vi "MQTT Transmitter (DBL).vi"() -> ()   [LabVIEW 2021]
uses:
  <vilib>/LabVIEW Open Source Project/MQTT Control Packets/Control Packets/CONNECT/ConnectFlags -- cluster.ctl
  <vilib>/LabVIEW Open Source Project/MQTT Client/Client class/Client.lvclass/Client.ctl
  <vilib>/LabVIEW Open Source Project/MQTT Client/Client class/Client.lvclass
  C:/Program Files (x86)/National Instruments/LabVIEW 2021/vi.lib/LabVIEW Open Source Project/MQTT Connection/MQTT_Base/Base Class/MQTT_Base.lvclass
  <vilib>/LabVIEW Open Source Project/Connection/Connection.TCP/Connection.TCP.lvclass
  C:/Program Files (x86)/National Instruments/LabVIEW 2021/vi.lib/LabVIEW Open Source Project/Connection/Connection/Connection.lvclass
  <vilib>/LabVIEW Open Source Project/MQTT Control Packets/Control Packets/PUBLISH/PUBLISH.lvclass
  <vilib>/LabVIEW Open Source Project/MQTT Connection/MQTT_Base/Base Class/MQTT_Base.lvclass
  <vilib>/LabVIEW Open Source Project/MQTT Control Packets/Control Packets/CONNECT/CONNECT.lvclass
panel:
  out "Published":bool
  in  "Send Topic":string="other/string"
  out "Send Chart":dbl(graph)
  out "Data Send":dbl format="%#_4g"
  in  "Time Target (s)":dbl=0.1 format="%#_6ps"
  out "Connected?":bool
  out "Read Chart":dbl(graph)
  out "Data Read":dbl format="%#_4g"
  in  "Read Topic":string="some/string"
  in  "remote port (1883)":u16=1883
  in  "address (localhost)":string="localhost"
  in  "STOP":bool
  # "MQTT Transmitter"
  # "Read"
  # "Send"
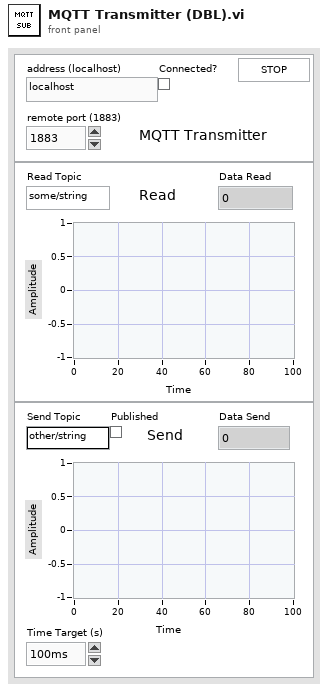
[diagram p1: front panel]
types:
  T1 = enum32{"Invalid", "Standard", "Closed", "Hidden", "Minimized", "Maximized"}
  T2 = enum32{"invalid app kind", "Development System", "Run Time System", "Student Edition", "Embedded LabVIEW", "Evaluation", "Custom"}
  T3 = cluster{"Will Topic":string, "Will Message":string, "Username":string, "Password":string}
  T4 = typedef "MQTT_Control_Packets.lvlib/CONNECT.lvclass/ConnectFlags -- cluster.ctl" = cluster{"Reserved":bool, "Clean Session":bool, "Will Flag":bool, "Will QoS 1":bool, "Will QoS 2":bool, "Will Retain":bool, "Password Flag":bool, "User Name Flag":bool}
  T5 = cluster{"Core":cluster{"Current VI Reference":refnum<vi>, "Close Panel on Exit?":bool}, "Connected?":bool, "Published?":bool, "Dummy Data":dbl}
  T6 = cluster{"Current VI Reference":refnum<vi>, "Close Panel on Exit?":bool}
  T7 = typedef "MQTT Client.lvlib/Client.lvclass/Public Events -- cluster.ctl" = cluster{"Connection Status":refnum<user-event>, "Connected":refnum<user-event>, "Application Message":refnum<user-event>}
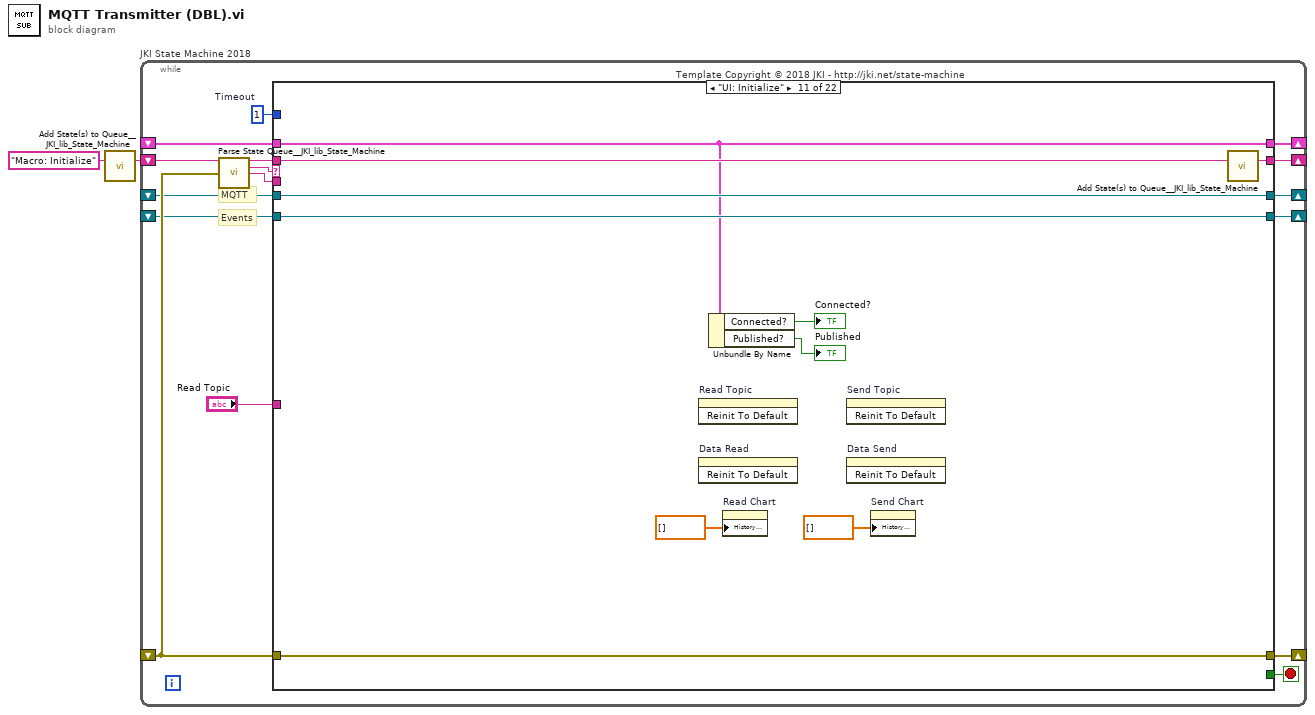
[diagram p0: block diagram]
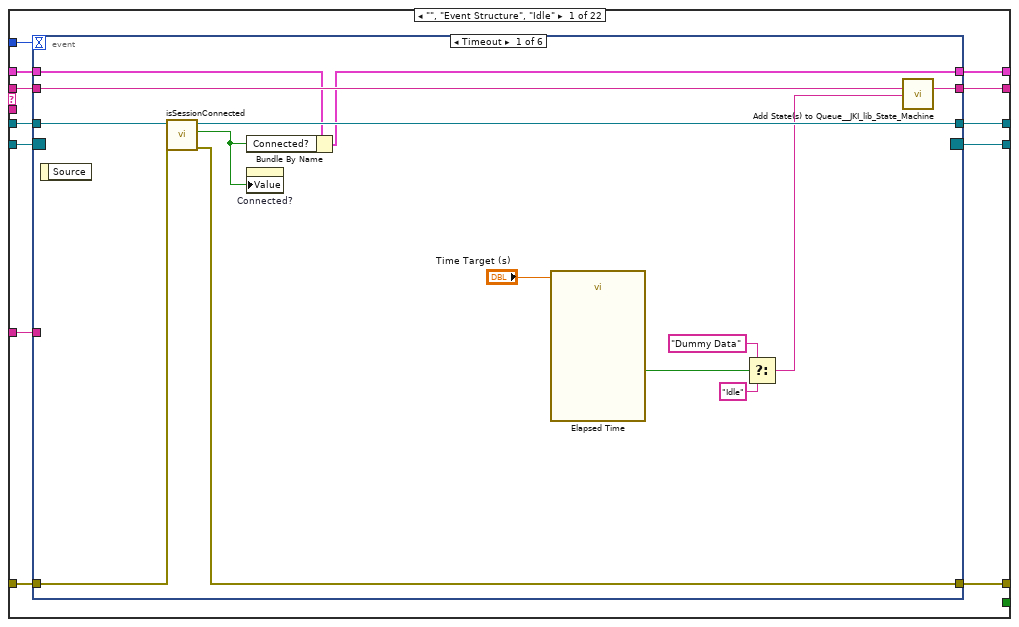
[diagram p2: hidden frame]
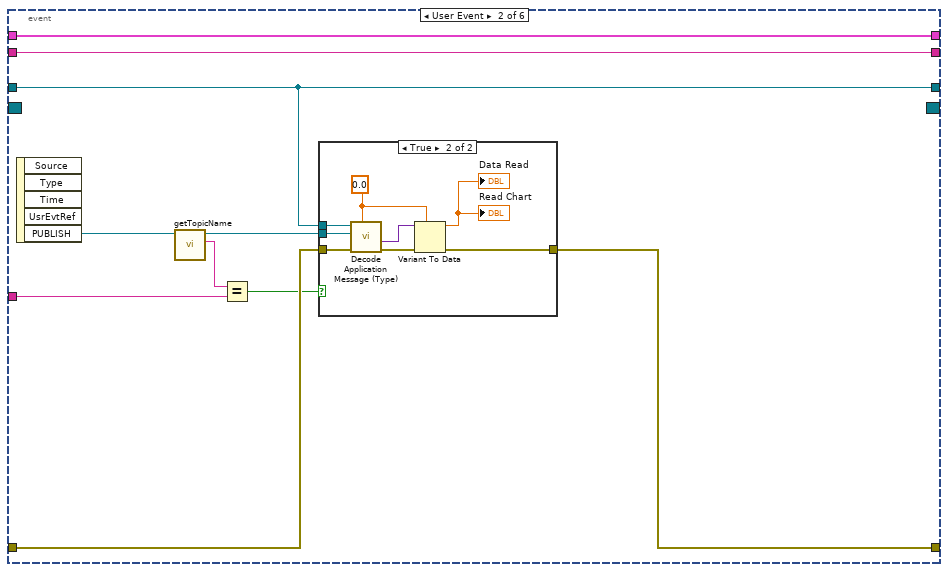
[diagram p3: hidden frame]
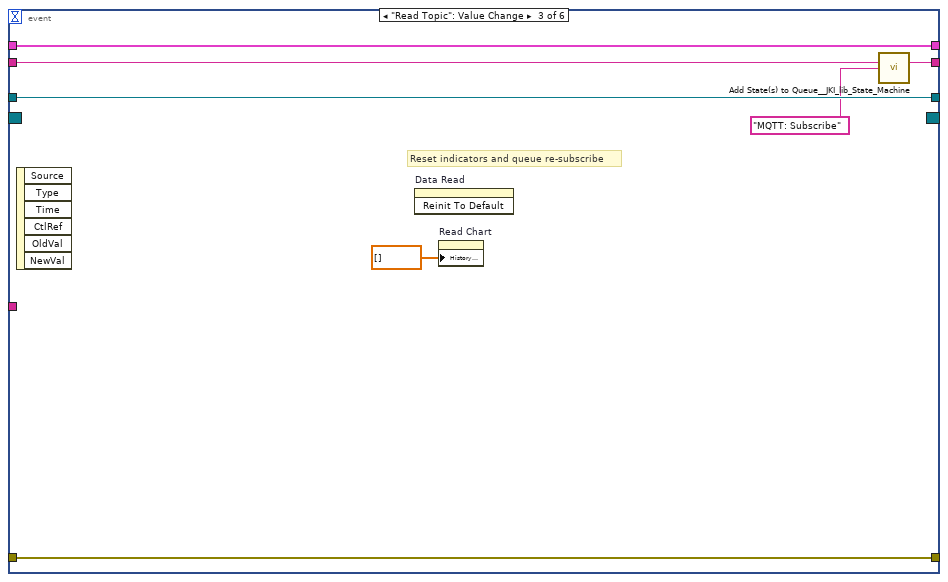
[diagram p5: hidden frame]
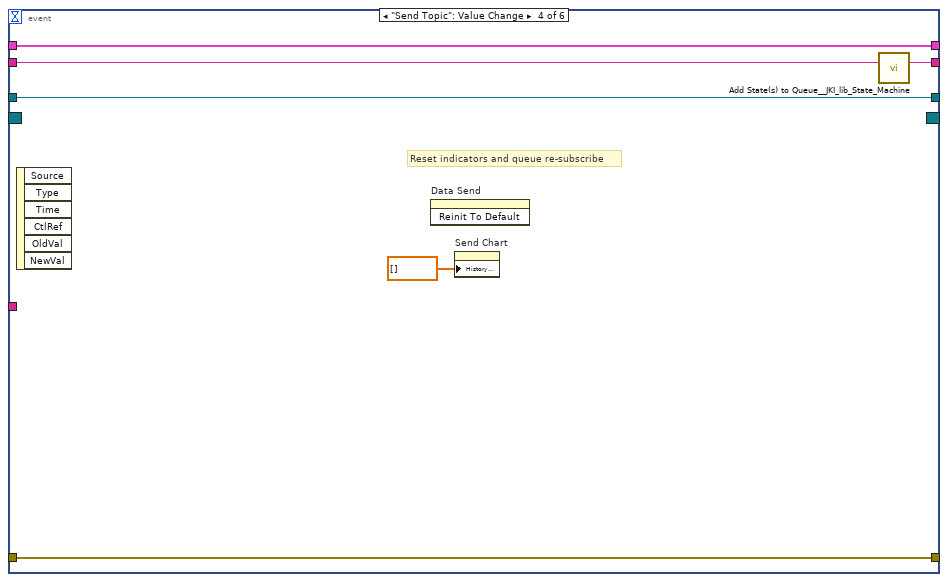
[diagram p6: hidden frame]
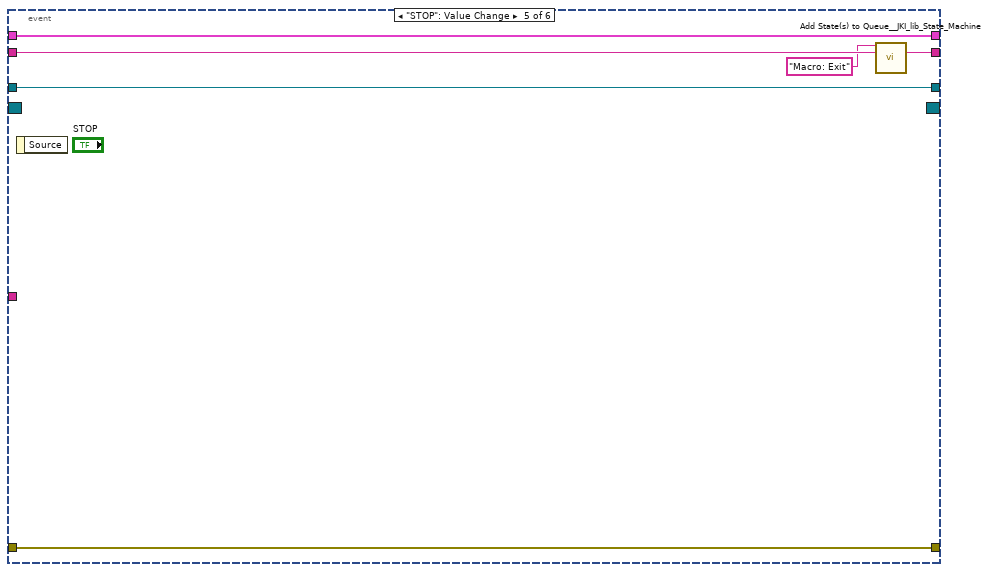
[diagram p7: hidden frame]
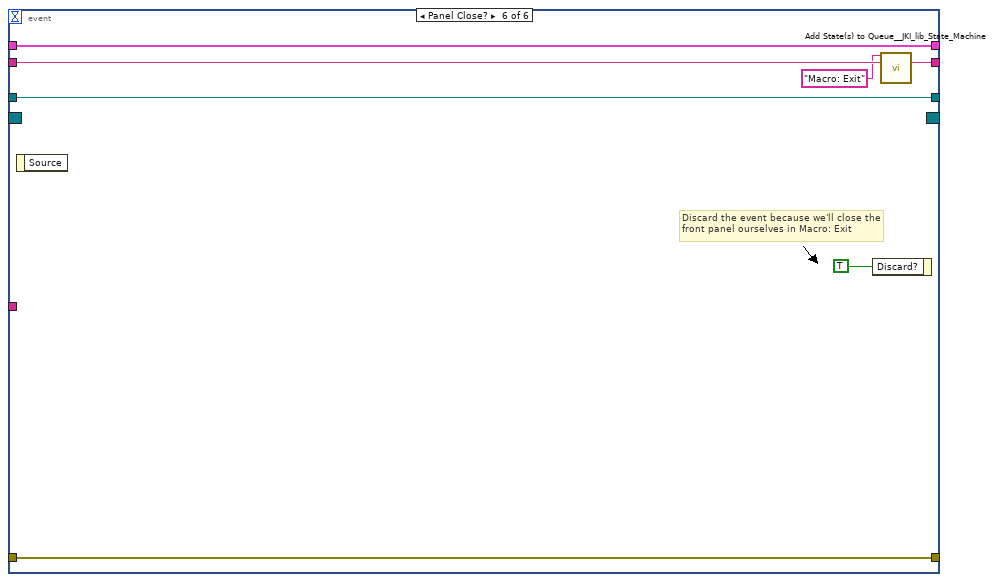
[diagram p8: hidden frame]
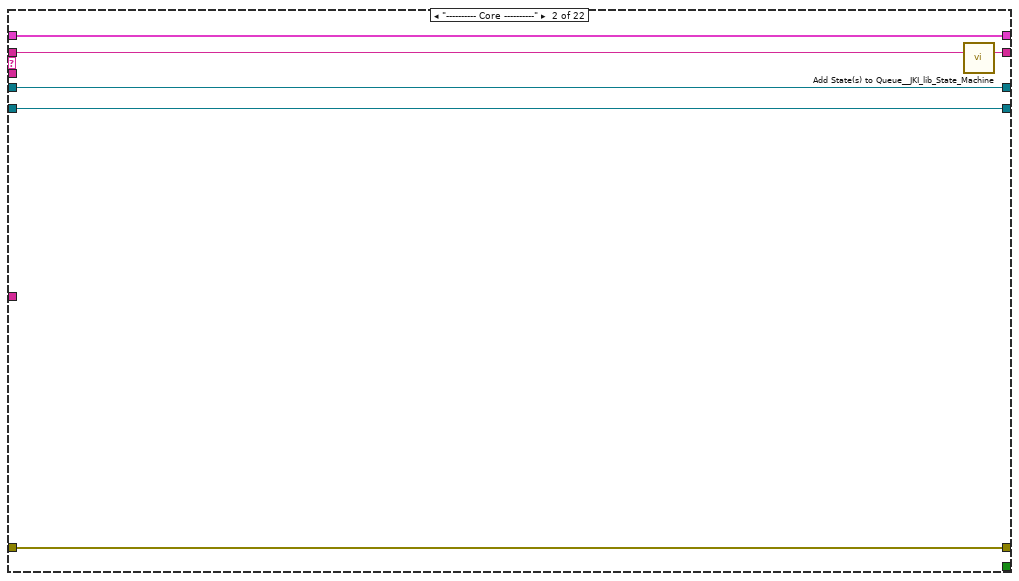
[diagram p9: hidden frame]
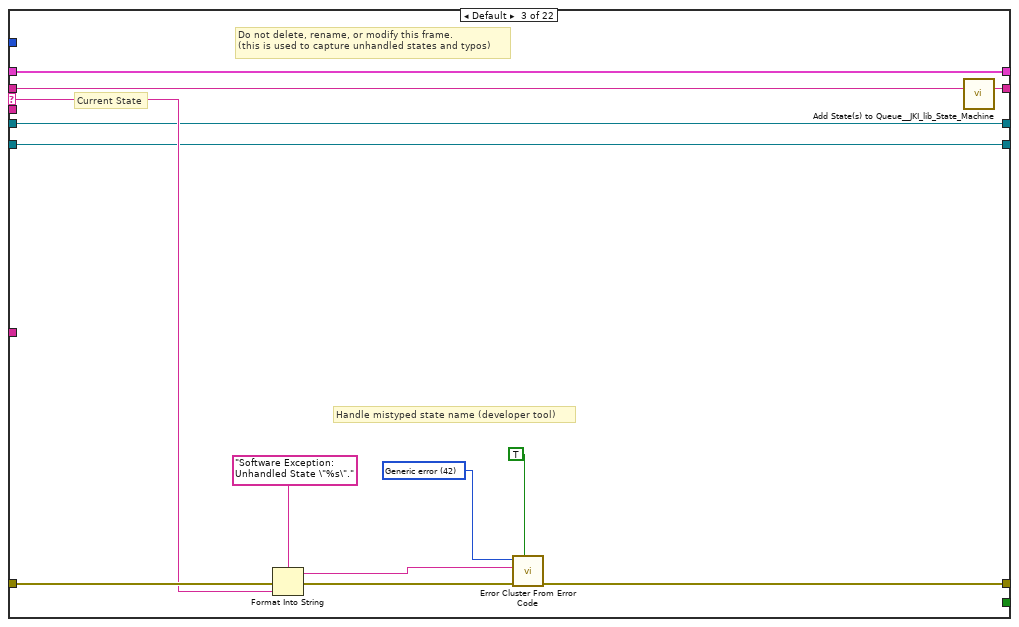
[diagram p10: hidden frame]
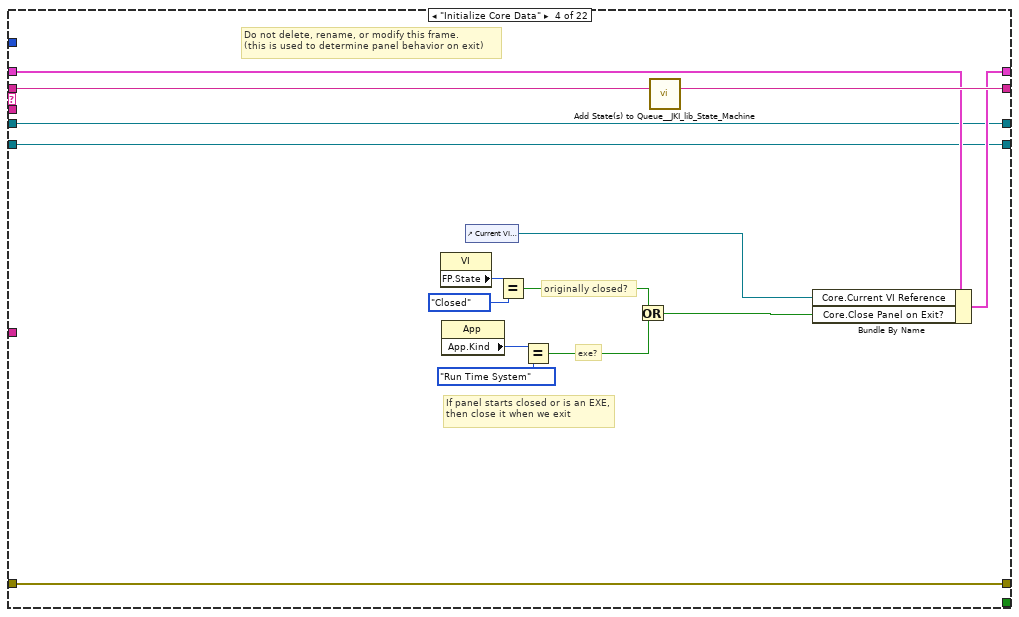
[diagram p11: hidden frame]
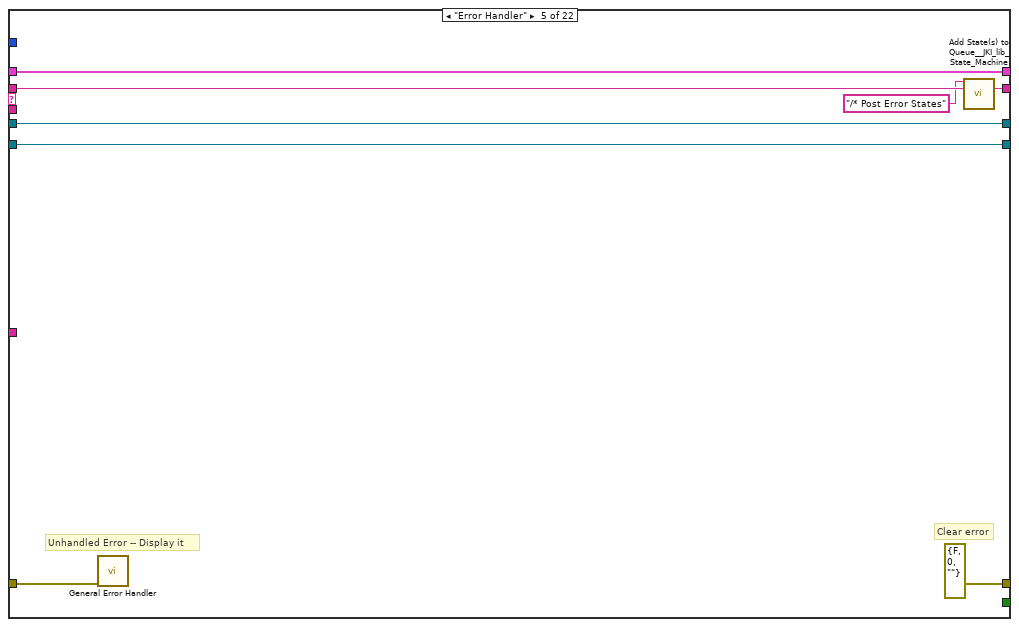
[diagram p12: hidden frame]
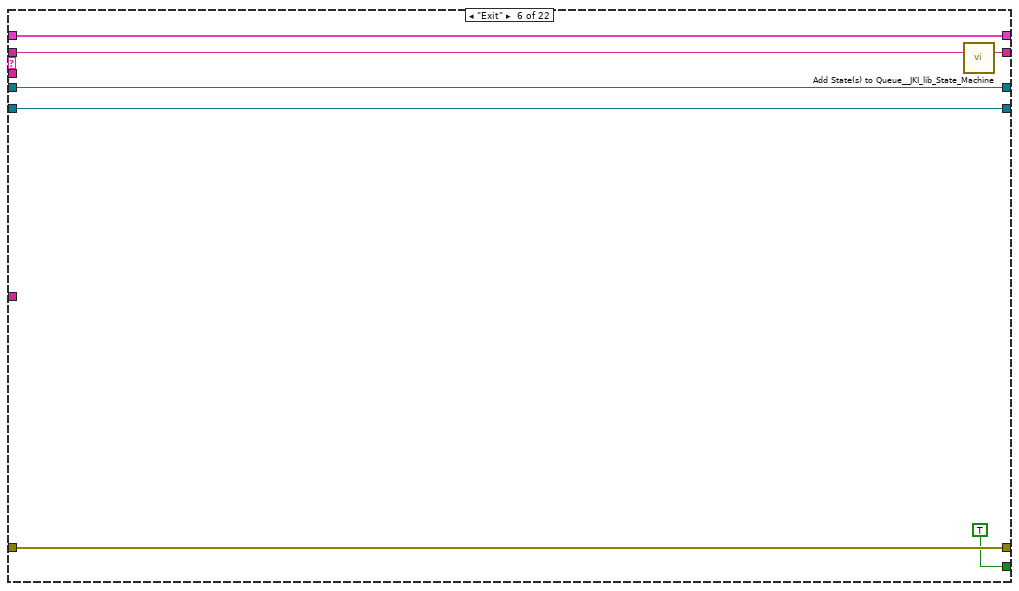
[diagram p13: hidden frame]
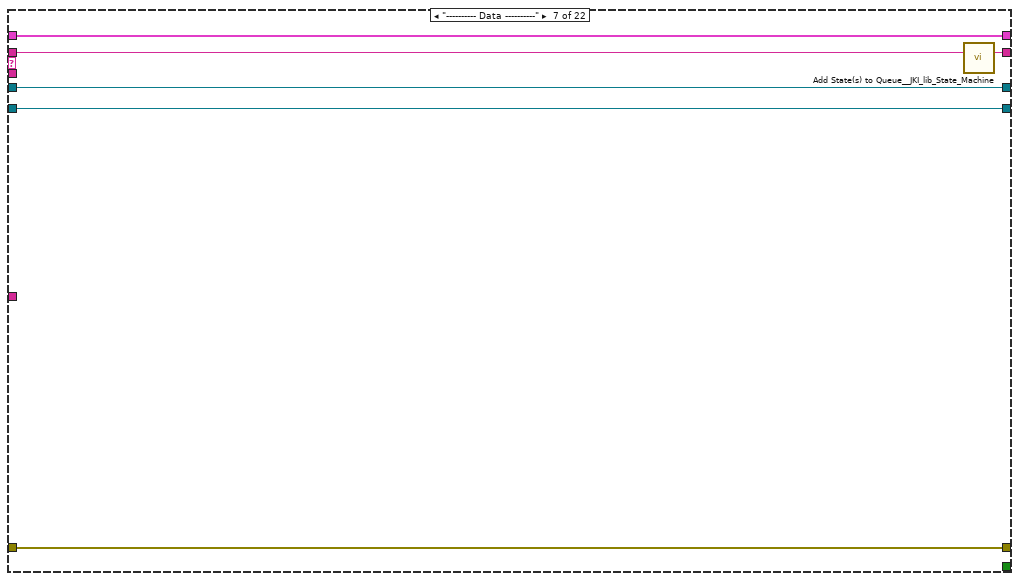
[diagram p14: hidden frame]
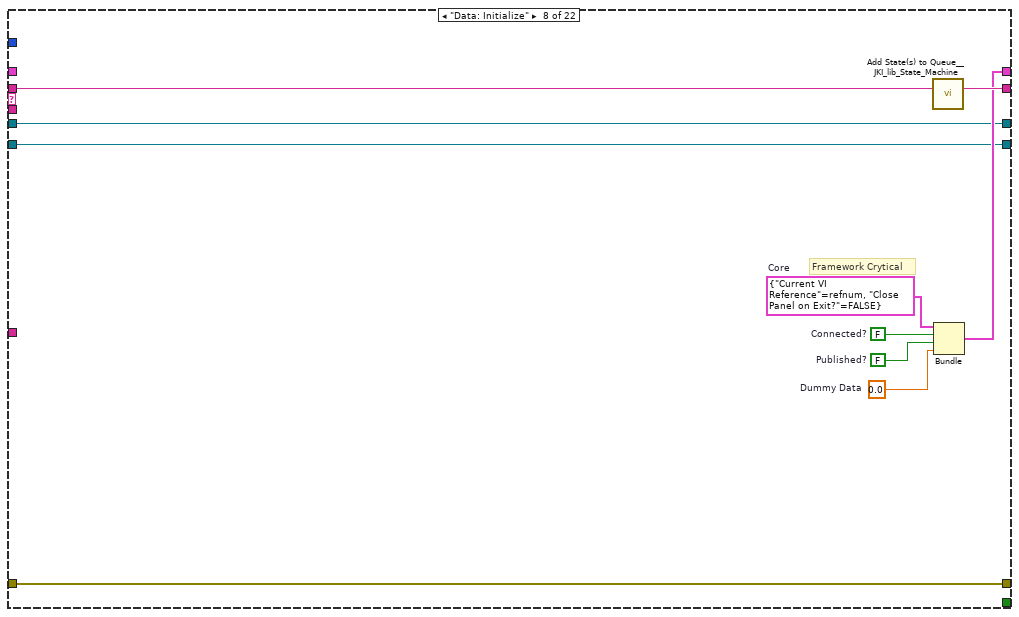
[diagram p15: hidden frame]
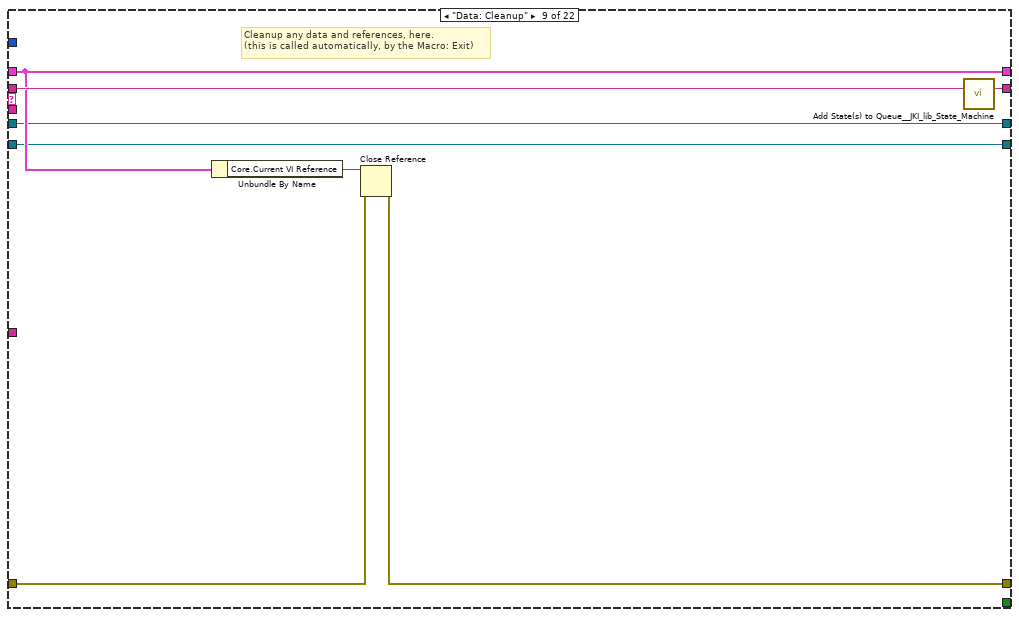
[diagram p16: hidden frame]
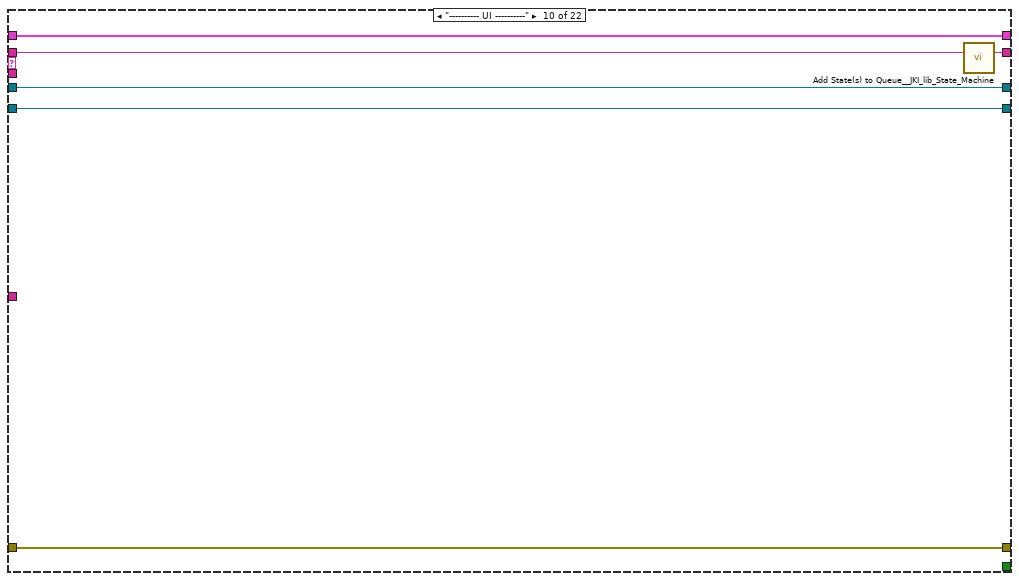
[diagram p17: hidden frame]
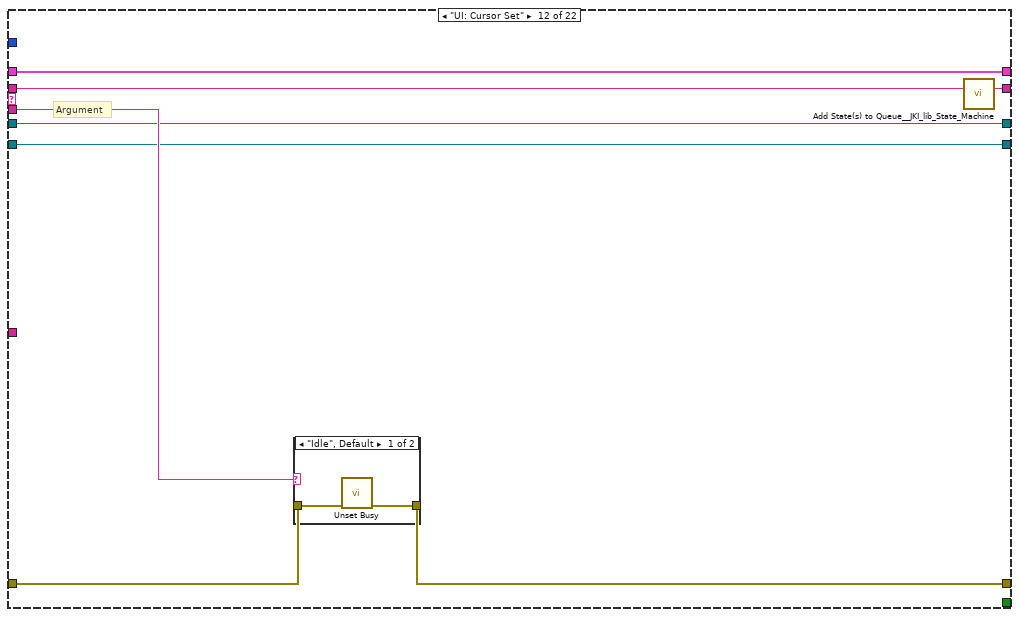
[diagram p18: hidden frame]
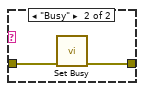
[diagram p19: hidden frame]
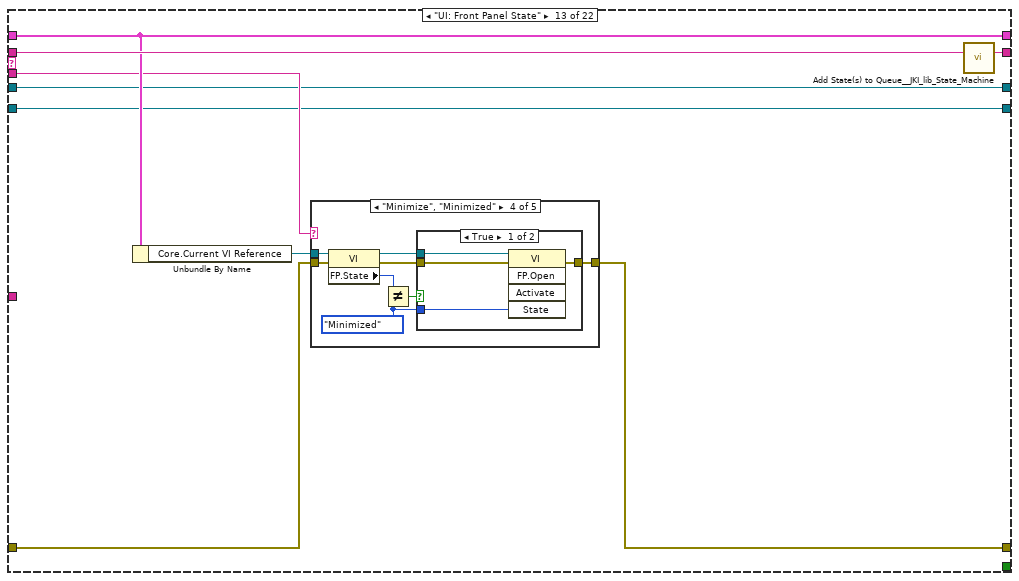
[diagram p20: hidden frame]
diagram:
  n1 = call <vilib>:"Add State(s) to Queue__JKI_lib_State_Machine.vi"("State(s) in (\"\")"="Macro: Initialize") -> ("States Out"=w2:string)  [unwired: 14 in]
  n2 = while "JKI State Machine 2018" {
    shift-right: [w11] -> _
    shift-left: _ -> [w10]
    shift-right: [w14] -> _
    shift-left: _ -> [w8]
    shift-right: [w13] -> _
    shift-left: w2 -> [w15]
    shift-right: [w7] -> _
    shift-left: _ -> [w6]
    shift-right: [w5] -> _
    shift-left: _ -> [w4]
    stop <- w12 stop-if-true
    w9 = 1  # Timeout
    # "Events"
    # "MQTT"
    # "Template Copyright © 2018 JKI - http://jki.net/state-machine"
    n3 = call <vilib>:"Parse State Queue__JKI_lib_State_Machine.vi"("State Queue"=w15, "Error In (no error)"=w8) -> ("Remaining States"=w17:string, "Current State"=w18:string, "Arguments"=w16:string)  [unwired: 11 in]
    n4 = case shown="\"UI: Initialize\"" w18 {
      selector: w18 -> [_ _ w98 _ _ _ _ _ _ _ _ _ _ _ _ _ _ _ _ _ _ _]
      tunnel: w17 -> [w30 w95 w102 w123 w131 w138 w144 w154 w162 w168 w178 w186 w199 w270 w277 w289 w295 w323 w325 w344 w364 w373]
      tunnel: w16 -> [_ _ _ _ _ _ _ _ _ _ _ w181 w193 _ _ _ _ _ _ _ _ _]
      tunnel: w10 -> [w28 w92 w100 w116 w128 w136 w141 _ w157 w165 w173 w184 w195 w267 w274 w286 w292 w303 w324 w342 w366 w371]
      tunnel: [w27 w93 w104 w120 errorcluster {"status"=FALSE, "code"=0, "source"=""} ("error out") w135 w142 w151 w158 w166 w176 w182 w196 w268 w275 w287 w293 w305 w326 w345 w365 w372] -> w14
      tunnel: w8 -> [w26 w93 w103 w120 w127 w135 w142 w151 w159 w166 w176 w183 w197 w268 w275 w287 w293 w321 w327 w348 w365 w372]
      tunnel: [w29 w94 w101 w122 w130 w137 w143 w153 w161 w167 w177 w185 w198 w269 w276 w288 w294 w322 w325 w344 w364 w375] -> w13
      tunnel: [_ _ _ _ _ TRUE _ _ _ _ _ _ _ _ _ _ _ _ _ _ _ _] -> w12
      tunnel: [w25 w92 w100 w121 w128 w136 w141 w152 w157 w165 w173 w184 w195 w267 w274 w286 w292 w302 w324 w343 w366 w370] -> w11
      tunnel: w9 -> [w24 _ _ _ _ _ _ _ _ _ _ _ _ _ _ _ _ _ _ _ _ _]
      tunnel: [w20 w90 w96 w109 w124 w132 w139 w147 w155 w163 w174 w179 w191 w265 w271 w278 w290 w320 w334 w353 w368 w378] -> w7
      tunnel: w6 -> [w21 w90 w96 w109 w124 w132 w139 w147 w155 w163 w174 w179 w191 w265 w271 w278 w290 _ w334 w353 w368 w378]
      tunnel: [w22 w91 w97 w110 w125 w133 w140 w148 w156 w164 w175 w180 w192 w266 w272 w279 w291 w304 w328 w346 w367 w377] -> w5
      tunnel: w4 -> [w23 w91 w97 w110 w125 w133 w140 w148 w156 w164 w175 w180 w192 w266 w272 w279 w291 _ w329 w347 w367 w377]
      tunnel: "Read Topic" -> [w19 _ _ _ _ _ _ _ _ _ _ _ _ _ _ _ _ _ w330 _ _ _]
      frame "", "Event Structure", "Idle" {
        n5 = event shown="[0] Timeout" {
          selector: w21 -> [_ _ _ _ _ _]
          dyn-events: [_ _ _ _ _ _] -> w20
          timeout: w24 -> [_ _ _ _ _ _]
          tunnel: w30 -> [w44 w54 w69 w75 w82 w89]
          tunnel: [w43 w54 w68 w74 w81 w88] -> w29
          tunnel: w28 -> [w38 w53 w70 w76 w79 w86]
          tunnel: [w39 w48 w67 w73 w80 w87] -> w27
          tunnel: w26 -> [w40 w49 w67 w73 w80 w87]
          tunnel: [w37 w53 w70 w76 w79 w86] -> w25
          tunnel: w23 -> [w42 w50 w66 w72 w77 w83]
          tunnel: [w41 w50 w66 w72 w77 w83] -> w22
          tunnel: w19 -> [_ w51 _ _ _ _]
          event Timeout {
            n6 = event-data() -> ()  [unwired: 1 in, 1 out]
            n7 = call <vilib>:"isSessionConnected.vi"("error in (no error)"=w40, "MQTT_Base in"=w42) -> ("error out"=w39:errorcluster, "Connected?"=w36:bool, "MQTT_Base out"=w41:refnum<class "Client.lvclass">)  [unwired: 7 in]
            n8 = Bundle By Name(cluster=w38, "Connected?"=w36) -> (w37:T5)
            n9 = property on="Connected?" class="Bool (strict)"("Value"=w36) -> ()  [unwired: 2 in, 2 out]
            n10 = call "Elapsed Time"("Time Target (s)"="Time Target (s)") -> ("Time has Elapsed"=w35:bool)  [unwired: 11 in, 7 out]
            n11 = Select(t="Dummy Data" ("State(s) at Back (\"\")"), s=w35, f="Idle" ("State(s) at Back (\"\")")) -> (s? t:f=w32:string)
            n12 = call <vilib>:"Add State(s) to Queue__JKI_lib_State_Machine.vi"("State(s) in (\"\")"=w44, "State(s) at Back (\"\")"=w32) -> ("States Out"=w43:string)  [unwired: 13 in]
          }
          event User Event {
            n13 = event-data() -> ("PUBLISH"=w52:refnum<class "PUBLISH.lvclass">)  [unwired: 1 in, 4 out]
            n14 = call <vilib>:"getTopicName.vi"("PUBLISH in"=w52) -> ("Topic"=w45:string, "PUBLISH out"=w46:refnum<class "PUBLISH.lvclass">)  [unwired: 8 in, 1 out]
            n15 = Equal?(x=w45, y=w51) -> (x = y?=w47:bool)
            n16 = case shown="True" w47 {
              tunnel: w50 -> [_ w63]
              tunnel: w49 -> [w55 w62]
              tunnel: [w55 w57] -> w48
              tunnel: w46 -> [_ w56]
              frame False {
              }
              frame True {
                w59 = 0.0
                n17 = call <vilib>:"Decode Application Message (Type).vi"("Type"=w59, "error in (no error)"=w62, "PUBLISH"=w56, "Client in"=w63) -> ("error out"=w60:errorcluster, "Payload"=w61:variant)  [unwired: 4 in, 2 out]
                n18 = Variant To Data(error in=w60, type=w59, Variant=w61) -> (data=→"Data Read" →"Read Chart":dbl, error out=w57:errorcluster)
              }
            }
          }
          event "Read Topic": Value Change {
            # "Reset indicators and queue re-subscribe"
            n19 = event-data() -> ()  [unwired: 1 in, 6 out]
            n20 = invoke on="Data Read" class="DigNum (strict)" method="Reinit To Default"() -> ()  [unwired: 3 in, 3 out]
            n21 = property on="Read Chart" class="WFChart (strict)"("History Data"=dbl[] []) -> ()  [unwired: 2 in, 2 out]
            n22 = call <vilib>:"Add State(s) to Queue__JKI_lib_State_Machine.vi"("State(s) in (\"\")"=w69, "State(s) at Back (\"\")"="MQTT: Subscribe" ("State(s) at Back (\"\")")) -> ("States Out"=w68:string)  [unwired: 13 in]
          }
          event "Send Topic": Value Change {
            # "Reset indicators and queue re-subscribe"
            n23 = event-data() -> ()  [unwired: 1 in, 6 out]
            n24 = invoke on="Data Send" class="DigNum (strict)" method="Reinit To Default"() -> ()  [unwired: 3 in, 3 out]
            n25 = property on="Send Chart" class="WFChart (strict)"("History Data"=dbl[] []) -> ()  [unwired: 2 in, 2 out]
            n26 = call <vilib>:"Add State(s) to Queue__JKI_lib_State_Machine.vi"("State(s) in (\"\")"=w75) -> ("States Out"=w74:string)  [unwired: 14 in]
          }
          event "STOP": Value Change {
            n27 = event-data() -> ()  [unwired: 1 in, 1 out]
            n28 = call <vilib>:"Add State(s) to Queue__JKI_lib_State_Machine.vi"("State(s) in Front (\"\")"="Macro: Exit", "State(s) in (\"\")"=w82) -> ("States Out"=w81:string)  [unwired: 13 in]
          }
          event Panel Close? {
            # "Discard the event because we'll close the front panel ourselves in Macro: Exit"
            n29 = event-data() -> ()  [unwired: 1 in, 1 out]
            n30 = event-data("Discard?"=TRUE) -> ()  [unwired: 1 in, 1 out]
            n31 = call <vilib>:"Add State(s) to Queue__JKI_lib_State_Machine.vi"("State(s) in Front (\"\")"="Macro: Exit", "State(s) in (\"\")"=w89) -> ("States Out"=w88:string)  [unwired: 13 in]
          }
        }
      }
      frame "---------- Core ----------" {
        n32 = call <vilib>:"Add State(s) to Queue__JKI_lib_State_Machine.vi"("State(s) in (\"\")"=w95) -> ("States Out"=w94:string)  [unwired: 14 in]
      }
      frame Default {
        w107 = 42 items=["No error", "Argument error", "Memory is full", "Out of zone", "End of file", "File already open", "Generic file I/O error", "File not found", "File permission error", "Disk is full", "Duplicate path", "Too many files open", "System feature not enabled", "Resource file not found", "Cannot add resource", "Resource not found", "Image not found", "Image memory error", "Pen does not exist", "Config type invalid", "Config token not found", "Config parse error", "Config memory error", "Bad external code format", "Bad external code offset", "External code not present", "Null window", "Destroy window error", "Null menu", "Print aborted", "Bad print record", "Print driver error", "Windows error during printing", "Memory error during printing", "Print dialog error", "Generic print error", "Invalid device refnum", "Device not found", "Device parameter error", "Device unit error", "Cannot open device", "Device call aborted", "Generic error", "Cancelled by user", "Object ID too low", "Object ID too high", "Object not in heap", "Unknown heap", "Unknown object (invalid DefProc)", "Unknown object (DefProc not in table)", "Message out of range", "Invalid (null) method", "Unknown message", "Manager call not supported", "Bad address", "Network operation in progress", "Network operation timed out", "Connection is busy", "Network attribute not supported", "Network error", "Address in use", "System out of memory", "Connection aborted", "Connection refused", "Not connected", "Already connected", "Connection closed", "Initialization error (interapplication manager)", "Bad occurrence", "Wait on unbound occurrence handler", "Occurrence queue overflow", "Datalog type conflict", "Unused", "Unrecognized type (interapplication manager)", "Memory corrupt", "Failed to make temporary DLL", "Old CIN version", "Drag socket not found", "Failed to load drop-object", "Failed to register OLE object", "Failed to release OLE object", "Format specifier type mismatch", "Unknown format specifier", "Too few format specifiers", "Too many format specifiers", "Scan failed", "Newer CIN version", "Error converting to variant", "Runtime menu error", "Password tampered", "Variant attribute not found", "Incompatible variant data type", "Event data is not available", "Event Store is not present", "Occurrence is not found", "Event Queue is not created", "Event info is not available", "Refnum passed is NULL", "Error retrieving Class GUID", "Error retrieving CoClass GUID", "Error retrieving TypeLib GUID.", "Bad built application magic bytes.", "Specific driver is different from the specific driver associated with the Logical Name.", "There is no session opened to the class driver.", "Max Error", "MAX - Error with config objects", "MAX - Error loading configuration", "MAX - Group not supported"]
        # "Current State"
        # "Do not delete, rename, or modify this frame.\n(this is used to capture unhandled states and typos)"
        # "Handle mistyped state name (developer tool)"
        n33 = Format Into String(format string="Software Exception: Unhandled State \"%s\"." ("message"), error in=w103, w98) -> (resulting string=w106:string, error out=w105:errorcluster)  [unwired: 1 in]
        n34 = call <vilib>:"Error Cluster From Error Code.vi"("show call chain? (False)"=TRUE, "error in (no error)"=w105, "error message (\"\")"=w106, "error code (0)"=w107) -> ("error out"=w104:errorcluster)  [unwired: 5 in]
        n35 = call <vilib>:"Add State(s) to Queue__JKI_lib_State_Machine.vi"("State(s) in (\"\")"=w102) -> ("States Out"=w101:string)  [unwired: 14 in]
      }
      frame "Initialize Core Data" {
        # "Do not delete, rename, or modify this frame.\n(this is used to determine panel behavior on exit)"
        # "originally closed?"
        # "exe?"
        # "If panel starts closed or is an EXE, then close it when we exit"
        n36 = property class="VI"() -> ("FP.State"=w113:T1)  [unwired: 2 in, 2 out]
        n37 = property class="App"() -> ("App.Kind"=w119:T2)  [unwired: 2 in, 2 out]
        n38 = control-ref of="Current VI Reference"() -> (w114:refnum<vi>)
        n39 = Equal?(x=w113, y=T1."Closed" ("Front Panel Window:State")) -> (x = y?=w111:bool)
        n40 = Equal?(x=w119, y=T2."Run Time System" ("Application:Kind")) -> (x = y?=w117:bool)
        n41 = Or(x=w111, y=w117) -> (x .or. y?=w115:bool)
        n42 = call <vilib>:"Add State(s) to Queue__JKI_lib_State_Machine.vi"("State(s) in (\"\")"=w123) -> ("States Out"=w122:string)  [unwired: 14 in]
        n43 = Bundle By Name(cluster=w116, "Core.Current VI Reference"=w114, "Core.Close Panel on Exit?"=w115) -> (w121:T5)
      }
      frame "Error Handler" {
        # "Unhandled Error -- Display it"
        # "Clear error"
        n44 = call <vilib>:"General Error Handler.vi"("error in (no error)"=w127) -> ()  [unwired: 10 in, 5 out]
        n45 = call <vilib>:"Add State(s) to Queue__JKI_lib_State_Machine.vi"("State(s) in Front (\"\")"="/* Post Error States", "State(s) in (\"\")"=w131) -> ("States Out"=w130:string)  [unwired: 13 in]
      }
      frame "Exit" {
        n46 = call <vilib>:"Add State(s) to Queue__JKI_lib_State_Machine.vi"("State(s) in (\"\")"=w138) -> ("States Out"=w137:string)  [unwired: 14 in]
      }
      frame "---------- Data ----------" {
        n47 = call <vilib>:"Add State(s) to Queue__JKI_lib_State_Machine.vi"("State(s) in (\"\")"=w144) -> ("States Out"=w143:string)  [unwired: 14 in]
      }
      frame "Data: Initialize" {
        w146 = FALSE  # Published?
        w145 = 0.0  # Dummy Data
        w149 = T6 {"Current VI Reference"=refnum, "Close Panel on Exit?"=FALSE}  # Core
        w150 = FALSE  # Connected?
        # "Framework Crytical"
        n48 = call <vilib>:"Add State(s) to Queue__JKI_lib_State_Machine.vi"("State(s) in (\"\")"=w154) -> ("States Out"=w153:string)  [unwired: 14 in]
        n49 = Bundle("Core"=w149, "Connected?"=w150, "Published?"=w146, "Dummy Data"=w145) -> (w152:T5)  [unwired: 1 in]
      }
      frame "Data: Cleanup" {
        # "Cleanup any data and references, here.\n(this is called automatically, by the Macro: Exit)"
        n50 = Unbundle By Name(w157) -> ("Core.Current VI Reference"=w160:refnum<vi>)
        n51 = Close Reference(reference=w160, error in (no error)=w159) -> (error out=w158:errorcluster)
        n52 = call <vilib>:"Add State(s) to Queue__JKI_lib_State_Machine.vi"("State(s) in (\"\")"=w162) -> ("States Out"=w161:string)  [unwired: 14 in]
      }
      frame "---------- UI ----------" {
        n53 = call <vilib>:"Add State(s) to Queue__JKI_lib_State_Machine.vi"("State(s) in (\"\")"=w168) -> ("States Out"=w167:string)  [unwired: 14 in]
      }
      frame "UI: Initialize" {
        n54 = invoke on="Read Topic" class="Str" method="Reinit To Default"() -> ()  [unwired: 3 in, 3 out]
        n55 = invoke on="Data Read" class="DigNum (strict)" method="Reinit To Default"() -> ()  [unwired: 3 in, 3 out]
        n56 = Unbundle By Name(w173) -> ("Connected?"=→"Connected?":bool, "Published?"=→"Published":bool)
        n57 = property on="Read Chart" class="WFChart (strict)"("History Data"=dbl[] []) -> ()  [unwired: 2 in, 2 out]
        n58 = invoke on="Send Topic" class="Str" method="Reinit To Default"() -> ()  [unwired: 3 in, 3 out]
        n59 = invoke on="Data Send" class="DigNum (strict)" method="Reinit To Default"() -> ()  [unwired: 3 in, 3 out]
        n60 = property on="Send Chart" class="WFChart (strict)"("History Data"=dbl[] []) -> ()  [unwired: 2 in, 2 out]
        n61 = call <vilib>:"Add State(s) to Queue__JKI_lib_State_Machine.vi"("State(s) in (\"\")"=w178) -> ("States Out"=w177:string)  [unwired: 14 in]
      }
      frame "UI: Cursor Set" {
        # "Argument"
        n62 = case shown="\"Idle\", Default" w181 {
          tunnel: w183 -> [w188 w190]
          tunnel: [w187 w189] -> w182
          frame "Idle", Default {
            n63 = call <vilib>:"Unset Busy.vi"("error in (no error)"=w188) -> ("error out"=w187:errorcluster)  [unwired: 10 in]
          }
          frame "Busy" {
            n64 = call <vilib>:"Set Busy.vi"("error in (no error)"=w190) -> ("error out"=w189:errorcluster)  [unwired: 9 in, 1 out]
          }
        }
        n65 = call <vilib>:"Add State(s) to Queue__JKI_lib_State_Machine.vi"("State(s) in (\"\")"=w186) -> ("States Out"=w185:string)  [unwired: 14 in]
      }
      frame "UI: Front Panel State" {
        n66 = Unbundle By Name(w195) -> ("Core.Current VI Reference"=w194:refnum<vi>)
        n67 = case shown="\"Minimize\", \"Minimized\"" w193 {
          tunnel: w197 -> [w205 w220 w231 w244 w257]
          tunnel: [w207 w221 w233 w246 w259] -> w196
          tunnel: w194 -> [w206 w218 w232 w245 w258]
          frame "Open", "Standard", Default {
            w200 = T1."Standard" ("State")
            n68 = property class="VI"(reference=w206, error in=w205) -> (reference out=w203:refnum<vi>, error out=w204:errorcluster, "FP.State"=w202:T1)
            n69 = Not Equal?(x=w202, y=w200) -> (x != y?=w201:bool)
            n70 = case shown="True" w201 {
              tunnel: [w211 w213] -> w207
              tunnel: w204 -> [w210 w213]
              tunnel: w203 -> [w209 _]
              tunnel: w200 -> [w208 _]
              frame True {
                n71 = invoke class="VI" method="FP.Open"(reference=w209, error in=w210, "Activate"=TRUE, "State"=w208) -> (error out=w211:errorcluster)  [unwired: 1 in, 4 out]
              }
              frame False {
              }
            }
          }
          frame "Close", "Closed" {
            n72 = property class="VI"(reference=w218, error in=w220) -> (reference out=w217:refnum<vi>, error out=w219:errorcluster, "FP.State"=w215:T1)
            n73 = Not Equal?(x=w215, y=T1."Closed" ("Front Panel Window:State")) -> (x != y?=w214:bool)
            n74 = case shown="True" w214 {
              tunnel: [w222 w225] -> w221
              tunnel: w219 -> [w222 w224]
              tunnel: w217 -> [_ w223]
              frame False {
              }
              frame True {
                n75 = invoke class="VI" method="FP.Close"(reference=w223, error in=w224) -> (error out=w225:errorcluster)  [unwired: 1 in, 2 out]
              }
            }
          }
          frame "Hidden", "Hide" {
            w226 = T1."Hidden" ("State")
            n76 = property class="VI"(reference=w232, error in=w231) -> (reference out=w229:refnum<vi>, error out=w230:errorcluster, "FP.State"=w228:T1)
            n77 = Not Equal?(x=w228, y=w226) -> (x != y?=w227:bool)
            n78 = case shown="True" w227 {
              tunnel: [w237 w238] -> w233
              tunnel: w230 -> [w236 w238]
              tunnel: w229 -> [w235 _]
              tunnel: w226 -> [w234 _]
              frame True {
                n79 = invoke class="VI" method="FP.Open"(reference=w235, error in=w236, "State"=w234) -> (error out=w237:errorcluster)  [unwired: 2 in, 4 out]
              }
              frame False {
              }
            }
          }
          frame "Minimize", "Minimized" {
            w239 = T1."Minimized" ("State")
            n80 = property class="VI"(reference=w245, error in=w244) -> (reference out=w242:refnum<vi>, error out=w243:errorcluster, "FP.State"=w241:T1)
            n81 = Not Equal?(x=w241, y=w239) -> (x != y?=w240:bool)
            n82 = case shown="True" w240 {
              tunnel: [w250 w251] -> w246
              tunnel: w243 -> [w249 w251]
              tunnel: w242 -> [w248 _]
              tunnel: w239 -> [w247 _]
              frame True {
                n83 = invoke class="VI" method="FP.Open"(reference=w248, error in=w249, "State"=w247) -> (error out=w250:errorcluster)  [unwired: 2 in, 4 out]
              }
              frame False {
              }
            }
          }
          frame "Maximize", "Maximized" {
            w252 = T1."Maximized" ("State")
            n84 = property class="VI"(reference=w258, error in=w257) -> (reference out=w255:refnum<vi>, error out=w256:errorcluster, "FP.State"=w254:T1)
            n85 = Not Equal?(x=w254, y=w252) -> (x != y?=w253:bool)
            n86 = case shown="True" w253 {
              tunnel: [w263 w264] -> w259
              tunnel: w256 -> [w262 w264]
              tunnel: w255 -> [w261 _]
              tunnel: w252 -> [w260 _]
              frame True {
                n87 = invoke class="VI" method="FP.Open"(reference=w261, error in=w262, "State"=w260) -> (error out=w263:errorcluster)  [unwired: 2 in, 4 out]
              }
              frame False {
              }
            }
          }
        }
        n88 = call <vilib>:"Add State(s) to Queue__JKI_lib_State_Machine.vi"("State(s) in (\"\")"=w199) -> ("States Out"=w198:string)  [unwired: 14 in]
      }
      frame "---------- Macro ----------" {
        n89 = call <vilib>:"Add State(s) to Queue__JKI_lib_State_Machine.vi"("State(s) in (\"\")"=w270) -> ("States Out"=w269:string)  [unwired: 14 in]
      }
      frame "Macro: Initialize" {
        n90 = call <vilib>:"Add State(s) to Queue__JKI_lib_State_Machine.vi"("State(s) in Front (\"\")"="Data: Initialize\nInitialize Core Data\nMQTT: Initialize\nUI: Initialize\nUI: Front Panel State >> Open", "State(s) in (\"\")"=w277) -> ("States Out"=w276:string)  [unwired: 13 in]
      }
      frame "Macro: Exit" {
        n91 = Unbundle By Name(w286) -> ("Core.Close Panel on Exit?"=w285:bool)
        n92 = Select(t="UI: Front Panel State >> Close", s=w285, f="") -> (s? t:f=w282:string)
        n93 = call <vilib>:"Add State(s) to Queue__JKI_lib_State_Machine.vi"("State(s) in (\"\")"=w282, "State(s) at Back (\"\")"="Data: Cleanup\nExit") -> ("States Out"=w280:string)  [unwired: 13 in]
        n94 = call <vilib>:"Add State(s) to Queue__JKI_lib_State_Machine.vi"("State(s) in Front (\"\")"=w280, "State(s) in (\"\")"=w289) -> ("States Out"=w288:string)  [unwired: 13 in]
      }
      frame "---------- MQTT Broker ----------" {
        n95 = call <vilib>:"Add State(s) to Queue__JKI_lib_State_Machine.vi"("State(s) in (\"\")"=w295) -> ("States Out"=w294:string)  [unwired: 14 in]
      }
      frame "MQTT: initialize" {
        # "Exit on fail"
        # "Connect"
        n96 = call <vilib>:"Configure TCP Connection.vi"("error in (no error)"=w321, "remote port (80)"="remote port (1883)", "address (localhost)"="address (localhost)") -> ("error out"=w316:errorcluster, "Connection.TCP"=w315:refnum<class "Connection.TCP.lvclass">)  [unwired: 7 in]
        n97 = call <vilib>:"Create MQTT Client.vi"("error in (no error)"=w316, "Connection Configuration"=w315) -> ("error out"=w313:errorcluster, "Client out"=w314:refnum<class "Client.lvclass">)  [unwired: 8 in]
        n98 = call <vilib>:"Read Public Events.vi"("error in (no error)"=w313, "Client in"=w314) -> ("error out"=w311:errorcluster, "Client Public Events"=w312:T7, "Client out"=w310:refnum<class "Client.lvclass">)  [unwired: 7 in]
        n99 = register-events(error in=w311, w312) -> (reference out=w320:refnum<event-registration>, error out=w319:errorcluster)  [unwired: 1 in]
        n100 = call <vilib>:"Start.vi"("error in (no error)"=w319, "MQTT_Base in"=w310) -> ("error out"=w308:errorcluster, "MQTT_Base out"=w309:refnum<class "Client.lvclass">)  [unwired: 7 in, 1 out]
        n101 = call <vilib>:"Connect to Server.vi"("Connect Flags"=T4 {"Reserved"=FALSE, "Clean Session"=TRUE, "Will Flag"=FALSE, "Will QoS 1"=FALSE, "Will QoS 2"=FALSE, "Will Retain"=FALSE, "Password Flag"=TRUE, "User Name Flag"=TRUE}, "Payload"=T3 {"Will Topic"="", "Will Message"="", "Username"="username", "Password"="password"}, "error in (no error)"=w308, "Client in"=w309) -> ("error out"=w306:errorcluster, "Client out"=w307:refnum<class "Client.lvclass">)  [unwired: 4 in, 2 out]
        n102 = call <vilib>:"isSessionConnected.vi"("error in (no error)"=w306, "MQTT_Base in"=w307) -> ("error out"=w305:errorcluster, "Connected?"=w299:bool, "MQTT_Base out"=w304:refnum<class "Client.lvclass">)  [unwired: 7 in]
        n103 = Select(t="MQTT: Subscribe", s=w299, f="Macro: Exit" ("State(s) at Back (\"\")")) -> (s? t:f=w298:string)
        n104 = Bundle By Name(cluster=w303, "Connected?"=w299) -> (w302:T5)
        n105 = call <vilib>:"Add State(s) to Queue__JKI_lib_State_Machine.vi"("State(s) in (\"\")"=w323, "State(s) at Back (\"\")"=w298) -> ("States Out"=w322:string)  [unwired: 13 in]
      }
      frame "MQTT: Subscribe" {
        n106 = call <vilib>:"isSessionConnected.vi"("error in (no error)"=w327, "MQTT_Base in"=w329) -> ("error out"=w332:errorcluster, "Connected?"=w331:bool, "MQTT_Base out"=w333:refnum<class "Client.lvclass">)  [unwired: 7 in]
        n107 = case shown="True" w331 {
          tunnel: w333 -> [w336 w341]
          tunnel: w332 -> [w335 w340]
          tunnel: [w335 w339] -> w326
          tunnel: [w336 w338] -> w328
          tunnel: w330 -> [_ w337]
          frame False {
          }
          frame True {
            n108 = call <vilib>:"Subscribe (Scalar).vi"("error in (no error)"=w340, "Topic Filter"=w337, "Client in"=w341) -> ("error out"=w339:errorcluster, "Client out"=w338:refnum<class "Client.lvclass">)  [unwired: 6 in, 1 out]
          }
        }
        n109 = property on="Connected?" class="Bool (strict)"("Value"=w331) -> ()  [unwired: 2 in, 2 out]
      }
      frame "MQTT: Publish Data" {
        n110 = call <vilib>:"isSessionConnected.vi"("error in (no error)"=w348, "MQTT_Base in"=w347) -> ("error out"=w351:errorcluster, "Connected?"=w350:bool, "MQTT_Base out"=w352:refnum<class "Client.lvclass">)  [unwired: 7 in]
        n111 = case shown="True" w350 {
          tunnel: w352 -> [w354 w362]
          tunnel: w351 -> [w355 w361]
          tunnel: w342 -> [_ w363]
          tunnel: [_ w359] -> w349
          tunnel: [w355 w358] -> w345
          tunnel: [w354 w357] -> w346
          frame False {
          }
          frame True {
            n112 = Unbundle By Name(w363) -> ("Dummy Data"=w360:dbl)
            n113 = call <vilib>:"Publish.vi"("error in (no error)"=w361, "Payload"=w360, "Topic Name (empty: Payload name)"="Send Topic", "Client in"=w362) -> ("error out"=w358:errorcluster, "Published"=w359:bool, "Client out"=w357:refnum<class "Client.lvclass">)  [unwired: 5 in]
          }
        }
        n114 = property on="Connected?" class="Bool (strict)"("Value"=w350) -> ()  [unwired: 2 in, 2 out]
        n115 = property on="Published" class="Bool (strict)"("Value"=w349) -> ()  [unwired: 2 in, 2 out]
        n116 = Bundle By Name(cluster=w342, "Connected?"=w350, "Published?"=w349) -> (w343:T5)
      }
      frame "---------- Dummy Data ----------" {
      }
      frame "Dummy Data" {
        # "Generate a sine wave"
        n117 = for {
          N: 1 -> [_]
          shift-right: [w380] -> _
          shift-left: _ -> [w381]
          tunnel: [w379] -> w369
          n118 = Add(x=0.2, y=w381) -> (x+y=w380:dbl)
          n119 = Sine(x=w380) -> (sin(x)=w379:dbl)
        }
        "Send Chart" <- w369
        "Data Send" <- w369
        n120 = Bundle By Name(cluster=w371, "Dummy Data"=w369) -> (w370:T5)
        n121 = call <vilib>:"Add State(s) to Queue__JKI_lib_State_Machine.vi"("State(s) in (\"\")"=w373, "State(s) at Back (\"\")"="MQTT: Publish Data" ("State(s) at Back (\"\")")) -> ("States Out"=w375:string)  [unwired: 13 in]
      }
    }
  }
